vi "Start Command.vi"(8 "error in (no error)":errorcluster, 10 "Robot Actors.lvlib:Command.lvlib:Command.lvclass":refnum<class "Command Actor.lvclass">, 11 "Command Processor in":refnum<class "Command Processor Actor.lvclass">) -> (0 "error out":errorcluster, 3 "Command Processor out":refnum<class "Command Processor Actor.lvclass">)   [LabVIEW 2014, in "Robot Actor Framework.lvlib" / "Command Processor Actor.lvlib" / "Command Processor Actor.lvclass"]
uses:
  Command Processor Actor.lvclass
  Command Actor/Command Actor Class/Command Actor.lvclass
  Command Processor Actor.lvclass/Command Processor Actor.ctl
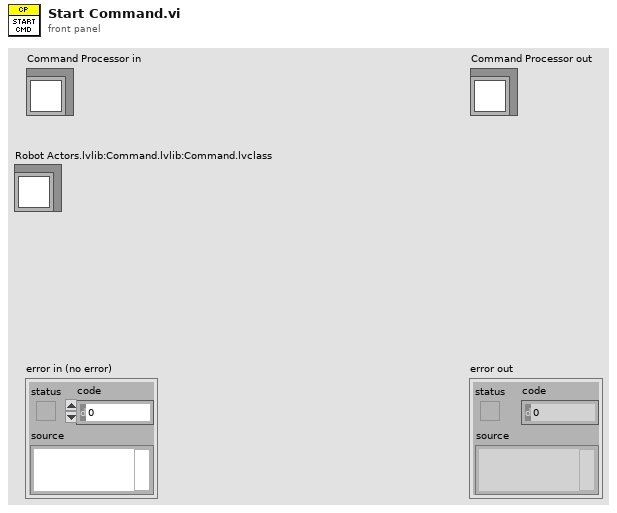
[diagram p1: front panel]
types:
  T1 = enum16{"Critical", "Error", "Warning", "Informational", "Debug"}
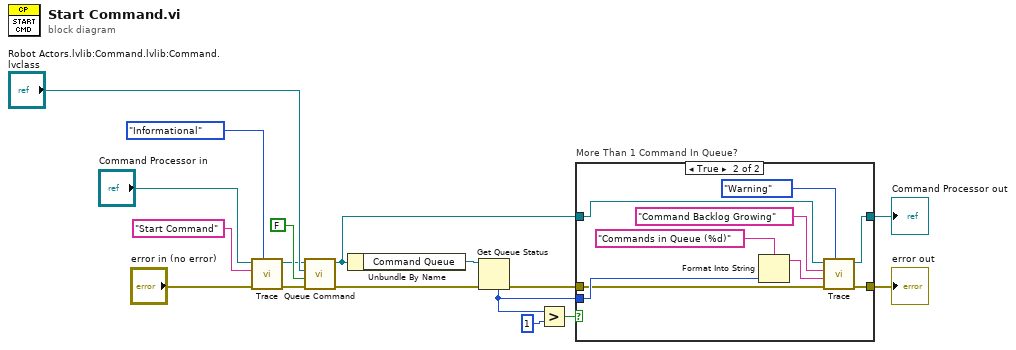
[diagram p0: block diagram]
diagram:
  n1 = call-dynamic "Trace.vi"("Trace Level"=T1."Informational", "error in (no error)"="error in (no error)", "Command Processor Action"="Start Command", "Command Processor Actor in"="Command Processor in") -> ("error out"=w11:errorcluster, "Command Processor Actor out"=w14:refnum<class "Command Processor Actor.lvclass">)  [unwired: 6 in]
  n2 = call-dynamic "Queue Command.vi"("error in (no error)"=w11, "Check Throttle"=FALSE, "Command in"="Robot Actors.lvlib:Command.lvlib:Command.lvclass", "Command Processor Actor in"=w14) -> ("error out"=w3:errorcluster, "Command Processor Actor out"=w5:refnum<class "Command Processor Actor.lvclass">)  [unwired: 4 in, 2 out]
  n3 = Unbundle By Name(w5) -> ("Command Queue"=w9:refnum<queue>)
  n4 = Get Queue Status(queue=w9, error in (no error)=w3) -> (error out=w2:errorcluster, # elements in queue=w6:i32)  [unwired: 1 in, 6 out]
  n5 = Greater?(x=w6, y=1) -> (0:w7:bool)
  n6 = case "More Than 1 Command In Queue?" shown="True" w7 {
    tunnel: w6 -> [_ w25]
    tunnel: w5 -> [w19 w24]
    tunnel: [w19 w23] -> w4
    tunnel: w2 -> [w18 w22]
    tunnel: [w18 w21] -> w1
    frame False {
    }
    frame True {
      n7 = Format Into String(format string="Commands in Queue (%d)", w25) -> (resulting string=w20:string)  [unwired: 2 in, 1 out]
      n8 = call-dynamic "Trace.vi"("Trace Level"=T1."Warning", "error in (no error)"=w22, "Command Processor Message"=w20, "Command Processor Action"="Command Backlog Growing", "Command Processor Actor in"=w24) -> ("error out"=w21:errorcluster, "Command Processor Actor out"=w23:refnum<class "Command Processor Actor.lvclass">)  [unwired: 5 in]
    }
  }
  "error out" <- w1
  "Command Processor out" <- w4
